vi "GetRobotPos.vi"(0 "Left Encoder":T1={"DevStatus"={"status"=FALSE, "code"=0, "source"=""}, "EncoderIndex"=enum."Invalid", "CounterIndex"=enum."Invalid", "DistancePerCount"=1.0, "Decoding Type"=enum."4x"}, 2 "X/Y/a In":T5, 3 "Right Encoder":T1={"DevStatus"={"status"=FALSE, "code"=0, "source"=""}, "EncoderIndex"=enum."Invalid", "CounterIndex"=enum."Invalid", "DistancePerCount"=1.0, "Decoding Type"=enum."4x"}) -> (6 "X/Y/a Out":T5)   [LabVIEW 2014]
uses:
  <vilib>/Rock Robotics/WPI/Encoder/WPI_EncoderDevRef.ctl
  <vilib>/Rock Robotics/SystemInterfaces/Encoder/FPGA_EncoderIdx.ctl
  <vilib>/Rock Robotics/SystemInterfaces/Counter/FPGA_CounterCtrSystemIndex.ctl
  <vilib>/Rock Robotics/WPI/Encoder/WPI_EncoderType.ctl
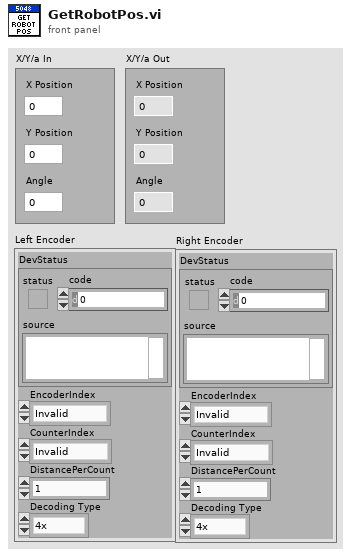
[diagram p1: front panel]
types:
  T1 = typedef "WPI_EncoderDevRef.ctl" = cluster{"DevStatus":errorcluster, "EncoderIndex":T2, "CounterIndex":T3, "DistancePerCount":dbl, "Decoding Type":T4}
  T2 = typedef "FPGA_EncoderIdx.ctl" = enum8{"Enc 0", "Enc 1", "Enc 2", "Enc 3", "Enc 4", "Enc 5", "Enc 6", "Enc 7", "Invalid"}
  T3 = typedef "FPGA_CounterCtrSystemIndex.ctl" = enum8{"Ctr 0", "Ctr 1", "Ctr 2", "Ctr 3", "Ctr 4", "Ctr 5", "Ctr 6", "Ctr 7", "Invalid"}
  T4 = typedef "WPI_EncoderType.ctl" = enum16{"1x", "2x", "4x"}
  T5 = cluster{"X Position":dbl, "Y Position":dbl, "Angle":dbl}
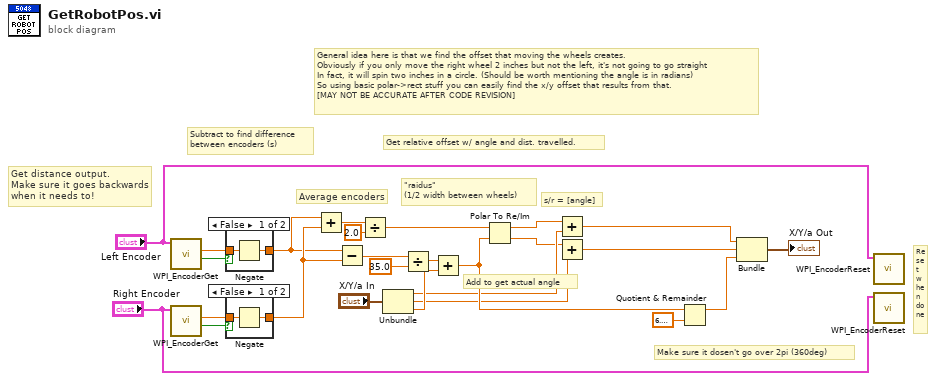
[diagram p0: block diagram]
diagram:
  # "Get relative offset w/ angle and dist. travelled."
  # "Average encoders"
  # "Add to get actual angle"
  # "Reset when done"
  # "Make sure it dosen't go over 2pi (360deg)"
  # "\"raidus\" \n(1/2 width between wheels)"
  # "s/r = [angle]"
  # "General idea here is that we find the offset that moving the wheels creates.\nObviously if you only move the right wheel 2 inches but not the left, it's not going to go straight\nIn fact, it will spin two inches in a circle. (Should be worth mentioning the angle is in radians)\nSo using basic polar->rect stuff you can easily find the x/y offset that results from that.\n[MAY NOT BE ACCURATE AFTER CODE REVISION]"
  # "Get distance output.\nMake sure it goes backwards\nwhen it needs to!"
  # "Subtract to find difference\nbetween encoders (s)"
  n1 = call <vilib>:"WPI_EncoderGet.vi"("EncoderDevRef"="Left Encoder") -> ("Direction"=w3:bool, "Distance"=w2:dbl)  [unwired: 5 in, 4 out]
  n2 = call <vilib>:"WPI_EncoderGet.vi"("EncoderDevRef"="Right Encoder") -> ("Direction"=w6:bool, "Distance"=w5:dbl)  [unwired: 5 in, 4 out]
  n3 = case shown="False" w3 {
    tunnel: w2 -> [w28 w29]
    tunnel: [w27 w29] -> w1
    frame False {
      n4 = Negate(x=w28) -> (-x=w27:dbl)
    }
    frame True {
    }
  }
  n5 = case shown="False" w6 {
    tunnel: w5 -> [w31 w32]
    tunnel: [w30 w32] -> w4
    frame False {
      n6 = Negate(x=w31) -> (-x=w30:dbl)
    }
    frame True {
    }
  }
  n7 = Add(x=w1, y=w4) -> (x+y=w16:dbl)
  n8 = Subtract(x=w1, y=w4) -> (x-y=w26:dbl)
  n9 = Divide(x=w16, y=2.0) -> (x/y=w14:dbl)
  n10 = Unbundle("X/Y/a In") -> ("X Position"=w11:dbl, "Y Position"=w9:dbl, "Angle"=w22:dbl)
  n11 = Divide(x=w26, y=35.0) -> (x/y=w24:dbl)
  n12 = Add(x=w24, y=w22) -> (x+y=w13:dbl)
  n13 = Polar To Re/Im(2:w13, 3:w14) -> (0:w10:dbl, 1:w12:dbl)
  n14 = Add(x=w12, y=w11) -> (x+y=w8:dbl)
  n15 = Add(x=w10, y=w9) -> (x+y=w7:dbl)
  n16 = Quotient & Remainder(x=w13, y=6.283185307179586) -> (x-y*floor(x/y)=w19:dbl)  [unwired: 1 out]
  n17 = Bundle(w8, w7, w19) -> (→"X/Y/a Out":cluster{dbl, dbl, dbl})  [unwired: 1 in]
  n18 = call <vilib>:"WPI_EncoderReset.vi"("EncoderDevRef"="Left Encoder") -> ()  [unwired: 9 in, 2 out]
  n19 = call <vilib>:"WPI_EncoderReset.vi"("EncoderDevRef"="Right Encoder") -> ()  [unwired: 9 in, 2 out]
